vi "FlatToRichnixnet_grpc_DbGetPropertyResponse.vi"(5 "OutputClusterType":T1, 11 "InputCluster":T2) -> (3 "OutputCluster":T1)   [LabVIEW 2025, in "grpc-xnet_client.lvlib"]
uses:
  grpc-xnet_client.lvlib
  nixnet_grpc_DbGetPropertyResponse_Flat.ctl
  nixnet_grpc_U32Array_Flat.ctl
  nidevice_grpc_Session_Flat.ctl
  nixnet_grpc_DbRefArray_Flat.ctl
  nixnet_grpc_DbGetPropertyResponse.ctl
  nixnet_grpc_DbGetPropertyResponse_property_value/nixnet_grpc_DbGetPropertyResponse_property_value.lvclass
  nixnet_grpc_DbGetPropertyResponse_property_value/nixnet_grpc_DbGetPropertyResponse_property_value.lvclass/nixnet_grpc_DbGetPropertyResponse_property_value.ctl
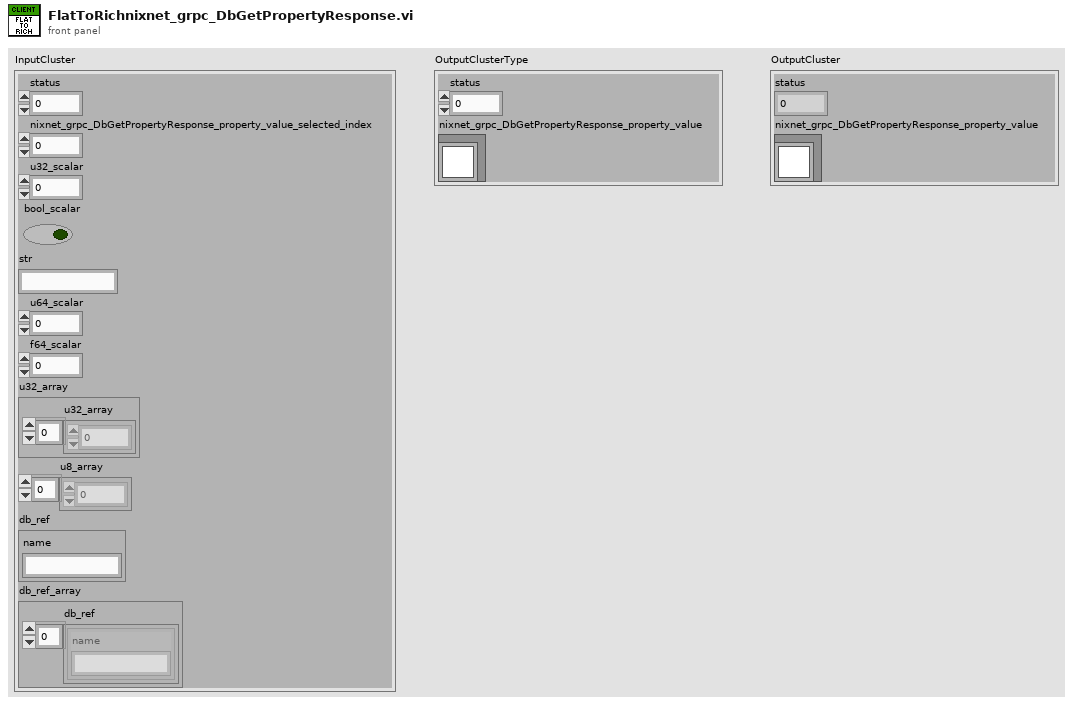
[diagram p1: front panel]
types:
  T1 = typedef "grpc-xnet_client.lvlib/nixnet_grpc_DbGetPropertyResponse.ctl" = cluster{"status":i32, "nixnet_grpc_DbGetPropertyResponse_property_value":refnum<class "nixnet_grpc_DbGetPropertyResponse_property_value.lvclass">}
  T2 = typedef "grpc-xnet_client.lvlib/nixnet_grpc_DbGetPropertyResponse_Flat.ctl" = cluster{"status":i32, "nixnet_grpc_DbGetPropertyResponse_property_value_selected_index":i32, "u32_scalar":u32, "bool_scalar":bool, "str":string, "u64_scalar":u64, "f64_scalar":dbl, "u32_array":T3, "u8_array":u8[], "db_ref":T4, "db_ref_array":T5}
  T3 = typedef "grpc-xnet_client.lvlib/nixnet_grpc_U32Array_Flat.ctl" = cluster{"u32_array":u32[]}
  T4 = typedef "grpc-xnet_client.lvlib/nidevice_grpc_Session_Flat.ctl" = cluster{"name":string}
  T5 = typedef "grpc-xnet_client.lvlib/nixnet_grpc_DbRefArray_Flat.ctl" = cluster{"db_ref":T4[]}
  T6 = typedef "grpc-xnet_client.lvlib/nixnet_grpc_U32Array.ctl" = cluster{"u32_array":u32[]}
  T7 = typedef "grpc-xnet_client.lvlib/nidevice_grpc_Session.ctl" = cluster{"name":string}
  T8 = typedef "grpc-xnet_client.lvlib/nixnet_grpc_DbRefArray.ctl" = cluster{"db_ref":T7[]}
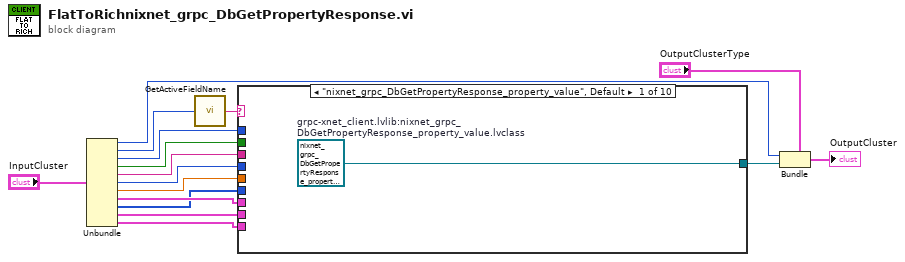
[diagram p0: block diagram]
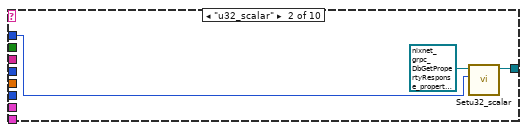
[diagram p2: hidden frame]
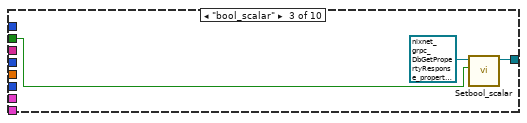
[diagram p3: hidden frame]
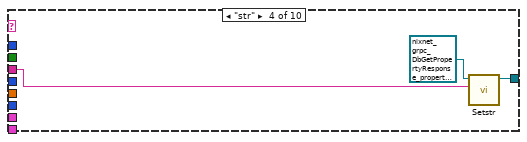
[diagram p4: hidden frame]
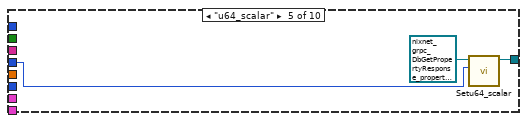
[diagram p5: hidden frame]
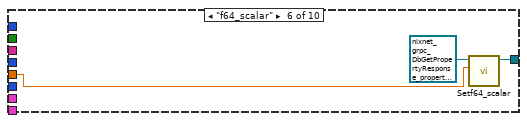
[diagram p6: hidden frame]
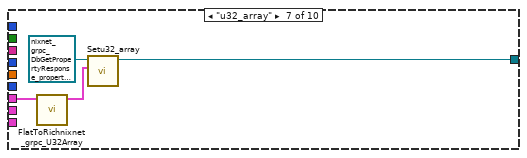
[diagram p7: hidden frame]
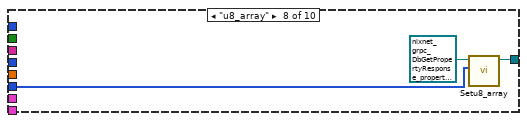
[diagram p8: hidden frame]
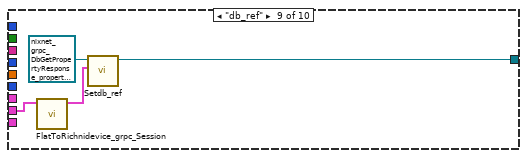
[diagram p9: hidden frame]
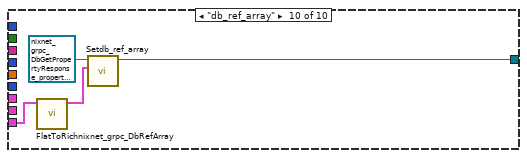
[diagram p10: hidden frame]
diagram:
  n1 = Unbundle "Unbundle"("InputCluster") -> ("status"=w13:i32, "nixnet_grpc_DbGetPropertyResponse_property_value_selected_index"=w12:i32, "u32_scalar"=w9:u32, "bool_scalar"=w8:bool, "str"=w7:string, "u64_scalar"=w6:u64, "f64_scalar"=w5:dbl, "u32_array"=w4:T3, "u8_array"=w3:u8[], "db_ref"=w2:T4, "db_ref_array"=w1:T5)
  n2 = call "GetActiveFieldName.vi"("protobuf index"=w12) -> ("oneof field name"=w11:string)
  n3 = case "nixnet_grpc_DbGetPropertyResponse_property_value" shown="\"nixnet_grpc_DbGetPropertyResponse_property_value\", Default" w11 {
    tunnel: [w17 w19 w22 w25 w28 w31 w34 w38 w41 w45] -> w10
    tunnel: w9 -> [_ w20 _ _ _ _ _ _ _ _]
    tunnel: w8 -> [_ _ w23 _ _ _ _ _ _ _]
    tunnel: w7 -> [_ _ _ w26 _ _ _ _ _ _]
    tunnel: w6 -> [_ _ _ _ w29 _ _ _ _ _]
    tunnel: w5 -> [_ _ _ _ _ w32 _ _ _ _]
    tunnel: w4 -> [_ _ _ _ _ _ w36 _ _ _]
    tunnel: w3 -> [_ _ _ _ _ _ _ w39 _ _]
    tunnel: w2 -> [_ _ _ _ _ _ _ _ w43 _]
    tunnel: w1 -> [_ _ _ _ _ _ _ _ _ w47]
    frame "nixnet_grpc_DbGetPropertyResponse_property_value", Default {
      w17 = refnum<class "nixnet_grpc_DbGetPropertyResponse_property_value.lvclass"> refnum  # grpc-xnet_client.lvlib:nixnet_grpc_DbGetPropertyResponse_property_value.lvclass
    }
    frame "u32_scalar" {
      n4 = call "Setu32_scalar.vi"("Set_Val"=w20, "OneOfTemplate in"=refnum<class "nixnet_grpc_DbGetPropertyResponse_property_value.lvclass"> refnum) -> ("OneOfTemplate out"=w19:refnum<class "nixnet_grpc_DbGetPropertyResponse_property_value.lvclass">)  [unwired: 8 in, 1 out]
    }
    frame "bool_scalar" {
      n5 = call "Setbool_scalar.vi"("Set_Val"=w23, "OneOfTemplate in"=refnum<class "nixnet_grpc_DbGetPropertyResponse_property_value.lvclass"> refnum) -> ("OneOfTemplate out"=w22:refnum<class "nixnet_grpc_DbGetPropertyResponse_property_value.lvclass">)  [unwired: 8 in, 1 out]
    }
    frame "str" {
      n6 = call "Setstr.vi"("Set_Val"=w26, "OneOfTemplate in"=refnum<class "nixnet_grpc_DbGetPropertyResponse_property_value.lvclass"> refnum) -> ("OneOfTemplate out"=w25:refnum<class "nixnet_grpc_DbGetPropertyResponse_property_value.lvclass">)  [unwired: 8 in, 1 out]
    }
    frame "u64_scalar" {
      n7 = call "Setu64_scalar.vi"("Set_Val"=w29, "OneOfTemplate in"=refnum<class "nixnet_grpc_DbGetPropertyResponse_property_value.lvclass"> refnum) -> ("OneOfTemplate out"=w28:refnum<class "nixnet_grpc_DbGetPropertyResponse_property_value.lvclass">)  [unwired: 8 in, 1 out]
    }
    frame "f64_scalar" {
      n8 = call "Setf64_scalar.vi"("Set_Val"=w32, "OneOfTemplate in"=refnum<class "nixnet_grpc_DbGetPropertyResponse_property_value.lvclass"> refnum) -> ("OneOfTemplate out"=w31:refnum<class "nixnet_grpc_DbGetPropertyResponse_property_value.lvclass">)  [unwired: 8 in, 1 out]
    }
    frame "u32_array" {
      n9 = call "FlatToRichnixnet_grpc_U32Array.vi"("InputCluster"=w36) -> ("OutputCluster"=w35:T6)  [unwired: 10 in]
      n10 = call "Setu32_array.vi"("Set_Val"=w35, "OneOfTemplate in"=refnum<class "nixnet_grpc_DbGetPropertyResponse_property_value.lvclass"> refnum) -> ("OneOfTemplate out"=w34:refnum<class "nixnet_grpc_DbGetPropertyResponse_property_value.lvclass">)  [unwired: 8 in, 1 out]
    }
    frame "u8_array" {
      n11 = call "Setu8_array.vi"("Set_Val"=w39, "OneOfTemplate in"=refnum<class "nixnet_grpc_DbGetPropertyResponse_property_value.lvclass"> refnum) -> ("OneOfTemplate out"=w38:refnum<class "nixnet_grpc_DbGetPropertyResponse_property_value.lvclass">)  [unwired: 8 in, 1 out]
    }
    frame "db_ref" {
      n12 = call "FlatToRichnidevice_grpc_Session.vi"("InputCluster"=w43) -> ("OutputCluster"=w42:T7)  [unwired: 10 in]
      n13 = call "Setdb_ref.vi"("Set_Val"=w42, "OneOfTemplate in"=refnum<class "nixnet_grpc_DbGetPropertyResponse_property_value.lvclass"> refnum) -> ("OneOfTemplate out"=w41:refnum<class "nixnet_grpc_DbGetPropertyResponse_property_value.lvclass">)  [unwired: 8 in, 1 out]
    }
    frame "db_ref_array" {
      n14 = call "FlatToRichnixnet_grpc_DbRefArray.vi"("InputCluster"=w47) -> ("OutputCluster"=w46:T8)  [unwired: 10 in]
      n15 = call "Setdb_ref_array.vi"("Set_Val"=w46, "OneOfTemplate in"=refnum<class "nixnet_grpc_DbGetPropertyResponse_property_value.lvclass"> refnum) -> ("OneOfTemplate out"=w45:refnum<class "nixnet_grpc_DbGetPropertyResponse_property_value.lvclass">)  [unwired: 8 in, 1 out]
    }
  }
  n16 = Bundle "Bundle"(cluster="OutputClusterType", "status"=w13, "nixnet_grpc_DbGetPropertyResponse_property_value"=w10) -> (→"OutputCluster":T1)
